vi "B-Spline Fit.vi"   [LabVIEW 2020, in "NI_AALPro.lvlib"]
doc: "Uses B-spline fitting to smooth a data set."
uses:
  <vilib>/Analysis/NI_AALPro.lvlib
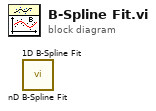
[diagram p0: block diagram]
diagram:
  n1 = call <vilib>:"nD B-Spline Fit.vi"() -> ()  [unwired: 13 in, 3 out]
  n2 = call <vilib>:"1D B-Spline Fit.vi"() -> ()  [unwired: 12 in, 4 out]
